vi "Vector 2D To SDL Point.vi"(11 "Vector 2D in":refnum<class "Vector 2D.lvclass">) -> (3 "Point":T1)   [LabVIEW 2021]
uses:
  LabSDL2/Source/Libraries/SDL2 Utility/Point (I32).ctl
  LabSDL2/Source/Libraries/SDL2 Utility/SDL2 Utility.lvlib
  Vector 2D/Vector 2D.lvclass
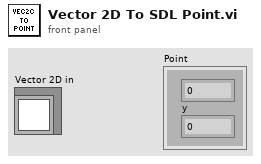
[diagram p1: front panel]
types:
  T1 = typedef "SDL2 Utility.lvlib/Point (I32).ctl" = cluster{"x":i32, "y":i32}
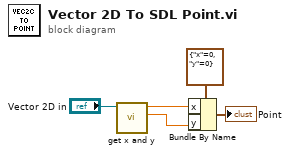
[diagram p0: block diagram]
diagram:
  n1 = call "get x and y.vi"("Vector 2D in"="Vector 2D in") -> ("y"=w2:sgl, "x"=w3:sgl)  [unwired: 9 in]
  n2 = Bundle By Name(cluster=T1 {"x"=0, "y"=0} ("Start"), "x"=w3, "y"=w2) -> (→"Point":T1)
